vi "TagContainer-ChangeDetector.vi"(8 "error in (no error)":errorcluster, 11 "TagContainer":T1) -> (0 "error out":errorcluster, 2 "Changed":bool, 3 "TagContainer(dup)":T1)   [LabVIEW 2017, in "TagContainer.lvlib"]
uses:
  TagContainer.lvlib
  Typedef/TagContainer.ctl
  4615f950-5bb4-4f5c-be7d-266d36556fe4.vi
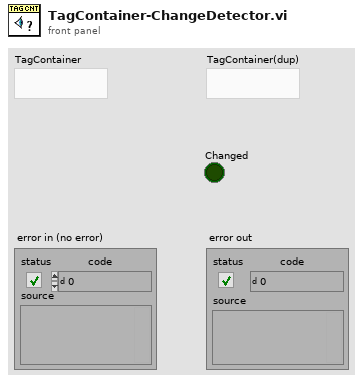
[diagram p1: front panel]
types:
  T1 = typedef "TagContainer.lvlib/TagContainer.ctl" = refnum<k1>
  T2 = typedef "TagContainer.lvlib/tagcontainer-data.ctl" = cluster{"tag-map":variant, "timestamp-map":variant, "namecacher-map":variant, "DataTypeCacher-map":variant, "Tag Adding Lock?":bool, "Global Change Timestamp":timestamp}
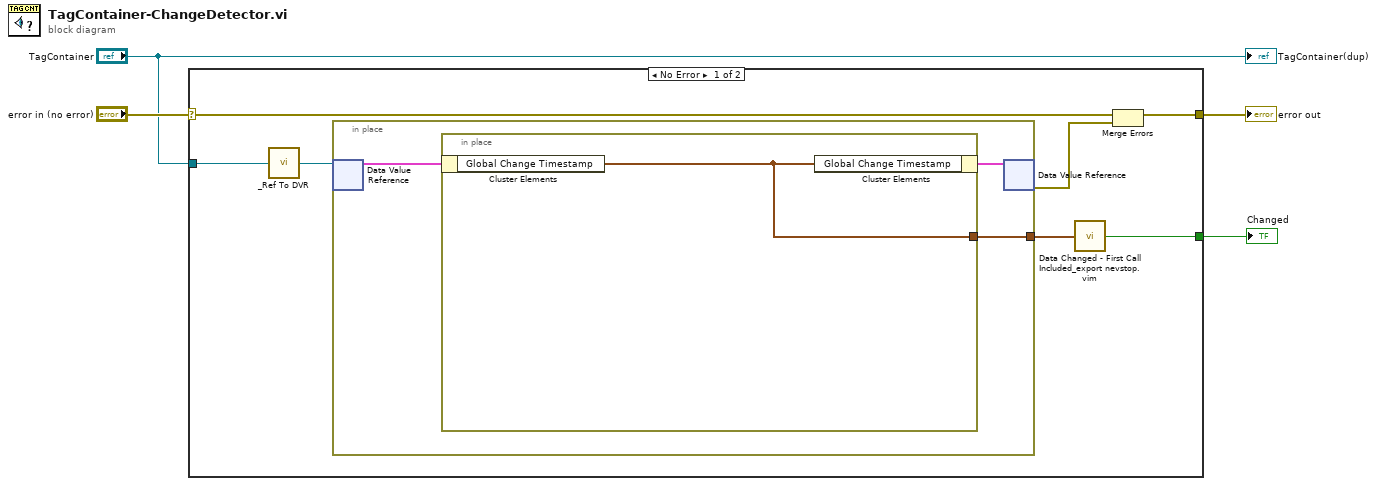
[diagram p0: block diagram]
diagram:
  n1 = case shown="No Error" "error in (no error)" {
    selector: "error in (no error)" -> [w10 w16]
    tunnel: [w11 w16] -> w3
    tunnel: "TagContainer" -> [w8 _]
    tunnel: [w5 _] -> w1
    frame No Error {
      n2 = call "_Ref To DVR.vi"("TagContainer"=w8) -> ("DVR"=w7:refnum<data-value>)
      n3 = in-place "In Place Element Structure" {
        in-place-border: [w12] -> w6
        n4 = in-place-dvr #1(w7) -> (w14:T2)  [unwired: 1 out]
        n5 = in-place {
          in-place-border: [w15] -> w12
          n6 = in-place-cluster #2(w14) -> ("Global Change Timestamp"=w15:timestamp)
          n7 = in-place-cluster #2("Global Change Timestamp"=w15) -> (w13:T2)
        }
        n8 = in-place-dvr #1(w13) -> (w9:errorcluster)  [unwired: 1 out]
      }
      n9 = call "Data Changed - First Call Included_export nevstop.vim"("Variant"=w6) -> ("Changed"=w5:bool)
      n10 = Merge Errors(w10, w9) -> (w11:errorcluster)
    }
    frame Error {
    }
  }
  "error out" <- w3
  "Changed" <- w1
  "TagContainer(dup)" <- "TagContainer"
